vi "Tektronix TDS 200 1000 2000 Series Acquire Multiple Waveforms.vi"() -> ()   [LabVIEW 2012]
doc: "This example shows how to configure multiple channels and acquire waveforms from multiple channels."
uses:
  <instrlib>/Tektronix TDS 200 1000 2000 Series/Public/Data/Read (Multiple Waveforms).vi
  <instrlib>/Tektronix TDS 200 1000 2000 Series/Tektronix TDS 200 1000 2000 Series.lvlib
panel:
  in  "Channel B (0: Channel 1)":u16(ring)=1 items=["Channel 1", "Channel 2", "Channel 3", "Channel 4", "Math", "Reference A", "Reference B", "Reference C", "Reference D"]
  in  "Channel A (0: Channel 1)":u16(ring) items=["Channel 1", "Channel 2", "Channel 3", "Channel 4", "Math", "Reference A", "Reference B", "Reference C", "Reference D"]
  in  "Serial Configuration":T1={"Baud Rate"=9600, "Parity"=0, "Stop Bits"=10, "Flow Control"=2} {"Flow Control" items=["None", "XON/XOFF", "RTS/CTS", "XON/XOFF & RTS/CTS", "DTR/DSR", "XON/XOFF & DTR/DSR"]; "Stop Bits" items=["1.0"=10, "1.5"=15, "2.0"=20]; "Parity" items=["None", "Odd", "Even", "Mark", "Space"]; "Baud Rate" items=["300"=300, "600"=600, "1200"=1200, "2400"=2400, "4800"=4800, "9600"=9600, "19200"=19200]}
  in  "Probe Attenuation B (1.0)":dbl=1.0
  in  "Vertical Coupling B (1: DC)":u16(ring)=1 items=["AC", "DC", "Ground"]
  in  "Probe Attenuation A (10.0)":dbl=10.0
  in  "Vertical Coupling A (1: DC)":u16(ring)=1 items=["AC", "DC", "Ground"]
  in  "Timeout (10000 ms)":u32=10000
  out "Waveform Data":waveform(dbl)[](graph)
  in  "VISA resource name":refnum<visa-resource-name>
  # "(C) 2009-2014 National Instruments.  ALL RIGHTS RESERVED."
  # "Channel A"
  # "Channel B"
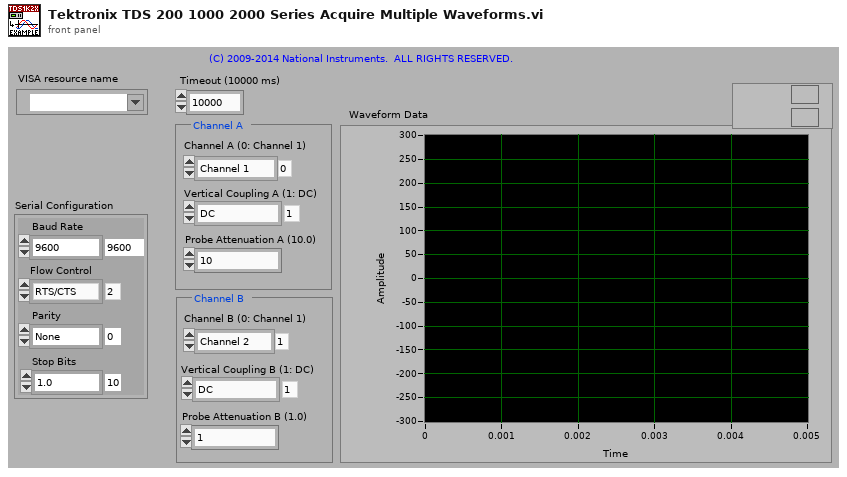
[diagram p1: front panel]
types:
  T1 = cluster{"Baud Rate":u32, "Parity":u16, "Stop Bits":u16, "Flow Control":u16}
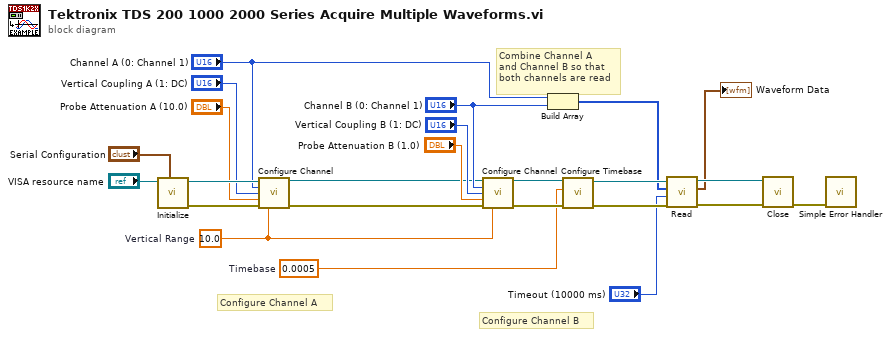
[diagram p0: block diagram]
diagram:
  w10 = 10.0  # Vertical Range
  w9 = 0.0005  # Timebase
  # "Combine Channel A\nand Channel B so that\nboth channels are read"
  # "Configure Channel B"
  # "Configure Channel A"
  n1 = call <instrlib>:"Initialize.vi"("Serial Configuration"="Serial Configuration", "VISA resource name"="VISA resource name") -> ("error out"=w19:errorcluster, "VISA resource name out"=w20:refnum<visa-resource-name>)  [unwired: 3 in, 5 out]
  n2 = call <instrlib>:"Configure Channel.vi"("VISA resource name"=w20, "Channel (0: Channel 1)"="Channel A (0: Channel 1)", "Vertical Coupling (1: DC)"="Vertical Coupling A (1: DC)", "Probe Attenuation (10: 10X)"="Probe Attenuation A (10.0)", "error in (no error)"=w19, "Vertical Range (10.0 V/div)"=w10) -> ("VISA resource name out"=w2:refnum<visa-resource-name>, "error out"=w1:errorcluster)  [unwired: 3 in, 5 out]
  n3 = call <instrlib>:"Configure Channel.vi"("VISA resource name"=w2, "Channel (0: Channel 1)"="Channel B (0: Channel 1)", "Vertical Coupling (1: DC)"="Vertical Coupling B (1: DC)", "Probe Attenuation (10: 10X)"="Probe Attenuation B (1.0)", "error in (no error)"=w1, "Vertical Range (10.0 V/div)"=w10) -> ("VISA resource name out"=w18:refnum<visa-resource-name>, "error out"=w17:errorcluster)  [unwired: 3 in, 5 out]
  n4 = Build Array("Channel A (0: Channel 1)", "Channel B (0: Channel 1)") -> (w6:u16[])
  n5 = call <instrlib>:"Configure Timebase.vi"("error in (no error)"=w17, "Timebase (0.0005 s)"=w9, "VISA resource name"=w18) -> ("error out"=w15:errorcluster, "VISA resource name out"=w16:refnum<visa-resource-name>)  [unwired: 1 in, 6 out]
  n6 = call-poly <instrlib>:"Read.vi"("error in (no error)"=w15, "Timeout (10000 ms)"="Timeout (10000 ms)", "Channels"=w6, "VISA resource name"=w16) -> ("error out"=w21:errorcluster, "Waveform Data"=→"Waveform Data":waveform(dbl)[], "VISA resource name out"=w22:refnum<visa-resource-name>)  [unwired: 5 out]
  n7 = call <instrlib>:"Close.vi"("error in (no error)"=w21, "VISA resource name"=w22) -> ("error out"=w23:errorcluster)  [unwired: 9 out]
  n8 = call <vilib>:"Simple Error Handler.vi"("error in (no error)"=w23) -> ()  [unwired: 1 in, 8 out]
